vi "Example.vi"() -> ()   [LabVIEW 2022 SP3]
uses:
  Source/VI-Snippet.lvlib
panel:
  out "Errot":errorcluster
  in  "Action":enum32{"Import VI Snippet", "Export VI Snippet"}(radio)
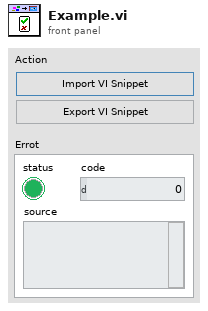
[diagram p1: front panel]
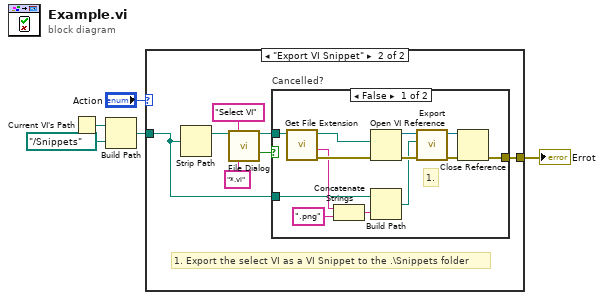
[diagram p0: block diagram]
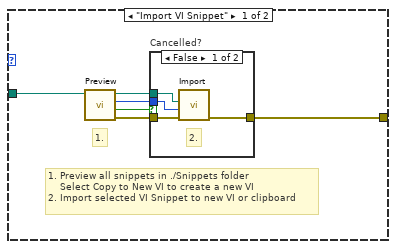
[diagram p2: hidden frame]
diagram:
  n1 = Current VI's Path() -> (path=w5:path)
  n2 = Build Path(base path=w5, name or relative path=path "../Snippets") -> (appended path=w3:path)
  n3 = case shown="\"Export VI Snippet\"" "Action" {
    tunnel: w3 -> [w11 w18]
    tunnel: [w6 w21] -> w1
    frame "Import VI Snippet" {
      # "1. Preview all snippets in ./Snippets folder\n    Select Copy to New VI to create a new VI \n2. Import selected VI Snippet to new VI or clipboard"
      # "1."
      n4 = call "Preview.vi"("VI Snippets Dir"=w11) -> ("error out"=w7:errorcluster, "Cancelled?"=w9:bool, "Copy to"=w10:enum8{"VI", "Clipboard"}, "VI Snippets Path"=w8:path)  [unwired: 7 in]
      n5 = case "Cancelled?" shown="False" w9 {
        tunnel: w10 -> [w13 _]
        tunnel: w8 -> [w14 _]
        tunnel: w7 -> [w15 w16]
        tunnel: [w12 w16] -> w6
        frame False {
          # "2."
          n6 = call "Import.vi"("error in (no error)"=w15, "Copy to (\"VI\")"=w13, "VI Snippet Path (.png)"=w14) -> ("error out"=w12:errorcluster)  [unwired: 6 in, 2 out]
        }
        frame True {
        }
      }
    }
    frame "Export VI Snippet" {
      # "1. Export the select VI as a VI Snippet to the .\\Snippets folder"
      n7 = Strip Path(path=w18) -> (stripped path=w17:path)  [unwired: 1 out]
      n8 = call "File Dialog"("start path"=w17, "prompt"="Select VI", "pattern (all files)"="*.vi") -> ("selected path"=w20:path, "cancelled"=w19:bool)  [unwired: 9 in, 2 out]
      n9 = case "Cancelled?" shown="False" w19 {
        tunnel: [w34 _] -> w21
        tunnel: w20 -> [w29 _]
        tunnel: w18 -> [w24 _]
        frame False {
          # "1."
          n10 = call <vilib>:"Get File Extension.vi"("file"=w29) -> ("error out"=w30:errorcluster, "filename without extension"=w26:string, "dup file"=w31:path)  [unwired: 6 in, 2 out]
          n11 = Concatenate Strings(w26, ".png" ("string")) -> (w27:string)
          n12 = Open VI Reference(vi path=w31, error in (no error)=w30) -> (vi reference=w33:refnum<vi>, error out=w36:errorcluster)  [unwired: 4 in]
          n13 = Build Path(base path=w24, name or relative path=w27) -> (appended path=w28:path)
          n14 = call "Export.vi"("error in (no error)"=w36, "VI Snippet Path (.png)"=w28, "VI Refnum"=w33) -> ("error out"=w35:errorcluster, "dup VI Refnum"=w32:refnum<vi>)  [unwired: 7 in]
          n15 = Close Reference(reference=w32, error in (no error)=w35) -> (error out=w34:errorcluster)
        }
        frame True {
        }
      }
    }
  }
  "Errot" <- w1
